vi "MOCKBEAR_Initialize.vi"(8 "error in (no error)":errorcluster, 11 "MOCKBEAR in":refnum<class "MOCKBEAR.lvclass">) -> (0 "error out":errorcluster, 3 "MOCKBEAR out":refnum<class "MOCKBEAR.lvclass">)   [LabVIEW 2021, in "MOCKBEAR.lvclass"]
uses:
  MOCKBEAR.lvclass
  MOCKBEAR.lvclass/MOCKBEAR.ctl
panel:
  out "error out 2":errorcluster caption="error out"
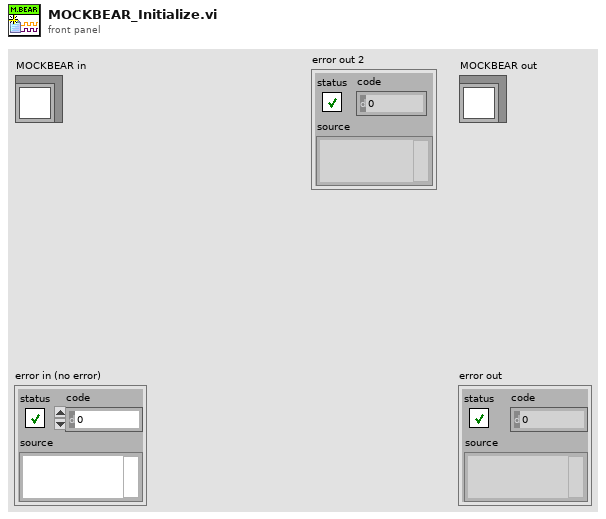
[diagram p1: front panel]
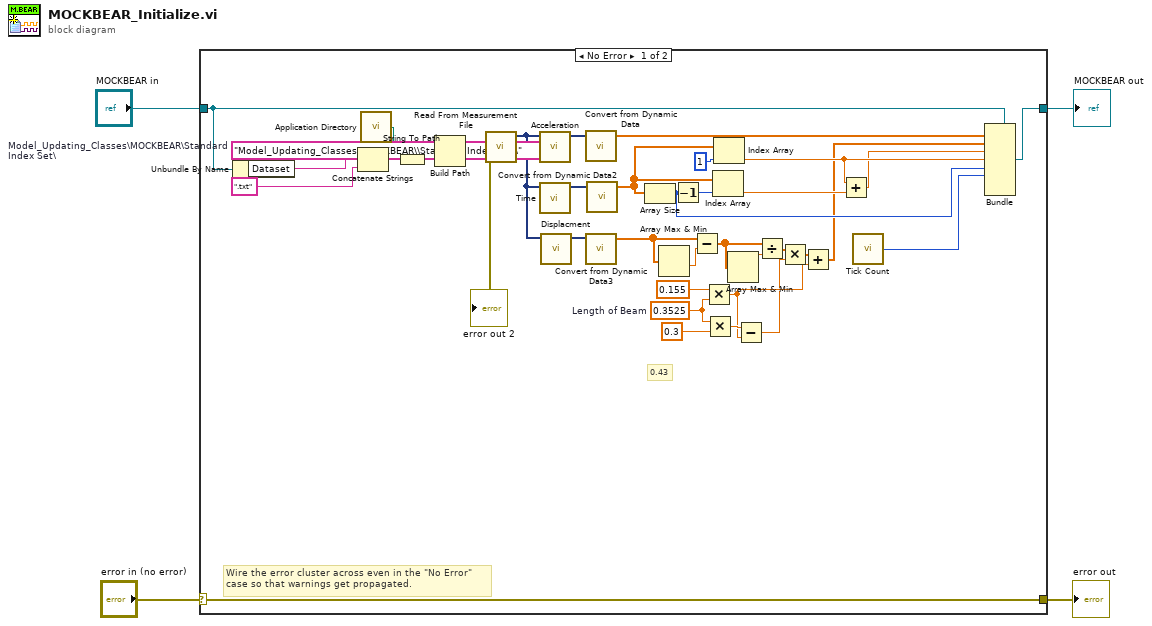
[diagram p0: block diagram]
diagram:
  n1 = case shown="No Error" "error in (no error)" {
    selector: "error in (no error)" -> [w41 w43]
    tunnel: [w41 w43] -> w3
    tunnel: [w11 w42] -> w1
    tunnel: "MOCKBEAR in" -> [w17 w42]
    frame No Error {
      w21 = "Model_Updating_Classes\\MOCKBEAR\\Standard Index Set\\"  # Model_Updating_Classes\MOCKBEAR\Standard Index Set\
      w30 = 0.3525  # Length of Beam
      # "0.43"
      # "Wire the error cluster across even in the \"No Error\"\ncase so that warnings get propagated."
      n2 = Unbundle By Name(w17) -> ("Dataset"=w20:string)
      n3 = Concatenate Strings(w21, w20, ".txt") -> (w22:string)
      n4 = call <vilib>:"Application Directory.vi"() -> ("Application Directory"=w9:path)
      n5 = String To Path(string=w22) -> (path=w18:path)
      n6 = Build Path(base path=w9, name or relative path=w18) -> (appended path=w40:path)
      n7 = call "Read From Measurement File"("Filename"=w40) -> ("error out"=→"error out 2":errorcluster, "Signals"=w33:dynamicdata)  [unwired: 5 in, 4 out]
      n8 = call "Acceleration"("Signals"=w33) -> ("Signal Out"=w38:dynamicdata)  [unwired: 9 in, 1 out]
      n9 = call "Time"("Signals"=w33) -> ("Signal Out"=w37:dynamicdata)  [unwired: 9 in, 1 out]
      n10 = call "Displacment"("Signals"=w33) -> ("Signal Out"=w32:dynamicdata)  [unwired: 9 in, 1 out]
      n11 = call "Convert from Dynamic Data"("Dynamic Data Type"=w38) -> ("Array"=w16:dbl[])  [unwired: 3 in]
      n12 = call "Convert from Dynamic Data3"("Dynamic Data Type"=w32) -> ("Array"=w26:dbl[])  [unwired: 3 in]
      n13 = call "Convert from Dynamic Data2"("Dynamic Data Type"=w37) -> ("Array"=w35:dbl[])  [unwired: 3 in]
      n14 = Array Size(array=w35) -> (size(s)=w12:i32)
      n15 = Array Max & Min(array=w26) -> (min value=w28:dbl)  [unwired: 3 out]
      n16 = Decrement(x=w12) -> (x-1=w34:i32)
      n17 = Subtract(x=w26, y=w28) -> (x-y=w25:dbl[])
      n18 = Multiply(x=0.155, y=w30) -> (x*y=w6:dbl)
      n19 = Multiply(x=w30, y=0.3) -> (x*y=w7:dbl)
      n20 = Index Array(array=w35, index=w34) -> (element=w39:dbl)
      n21 = Index Array(array=w35, index=1) -> (element=w15:dbl)
      n22 = Array Max & Min(array=w25) -> (max value=w24:dbl)  [unwired: 3 out]
      n23 = Subtract(x=w7, y=w6) -> (x-y=w5:dbl)
      n24 = Divide(x=w25, y=w24) -> (x/y=w23:dbl[])
      n25 = Multiply(x=w23, y=w5) -> (x*y=w27:dbl[])
      n26 = Add(x=w27, y=w6) -> (x+y=w8:dbl[])
      n27 = Add(x=w15, y=w39) -> (x+y=w14:dbl)
      n28 = call "Tick Count"() -> ("Tick Count(uSec)"=w13:u32)
      n29 = Bundle(cluster=w17, w16, w8, w14, w15, w12, w13) -> (w11:refnum<class "MOCKBEAR.lvclass">)  [unwired: 3 in]
    }
    frame Error {
    }
  }
  "error out" <- w3
  "MOCKBEAR out" <- w1
